vi "AcquisitionInterface1.vi"() -> ()   [LabVIEW 2025]
uses:
  <vilib>/DAQmx/read.llb/DAQmx Read (Analog 1D Wfm NChan NSamp).vi
  <vilib>/Waveform/WDTOps.llb/WDT Append Waveforms DBL.vi
panel:
  out "file path out":path
  in  "file path in":path
  out "error out":errorcluster
  in  "Save to txt":bool
  in  "stop":bool
  out "data":waveform(dbl)[](graph)
  in  "error in":errorcluster
  in  "physical channels":tag
  in  "channel settings":T1={"units"=10348, "input terminal configuration"=-1, "maximum value"=5.0, "minimum value"=-5.0} {"units" items=["Volts"=10348, "From Custom Scale"=10065]; "input terminal configuration" items=["Default"=-1, "RSE"=10083, "NRSE"=10078, "Differential"=10106, "Pseudodifferential"=12529]}
  in  "frequency settings":T2={"frequency (Hz)"=0.001, "number of samples per cycle"=2.0, "number of cycles"=1.0} {"frequency (Hz)" min=0.001 max=100000000.0; "number of samples per cycle" min=2.0 step=1.0; "number of cycles" min=1.0}
  # "Pulsa este botón para que la señal medida se guarde en un archivo .txt"
  # "Ruta en la que se guardará la señal"
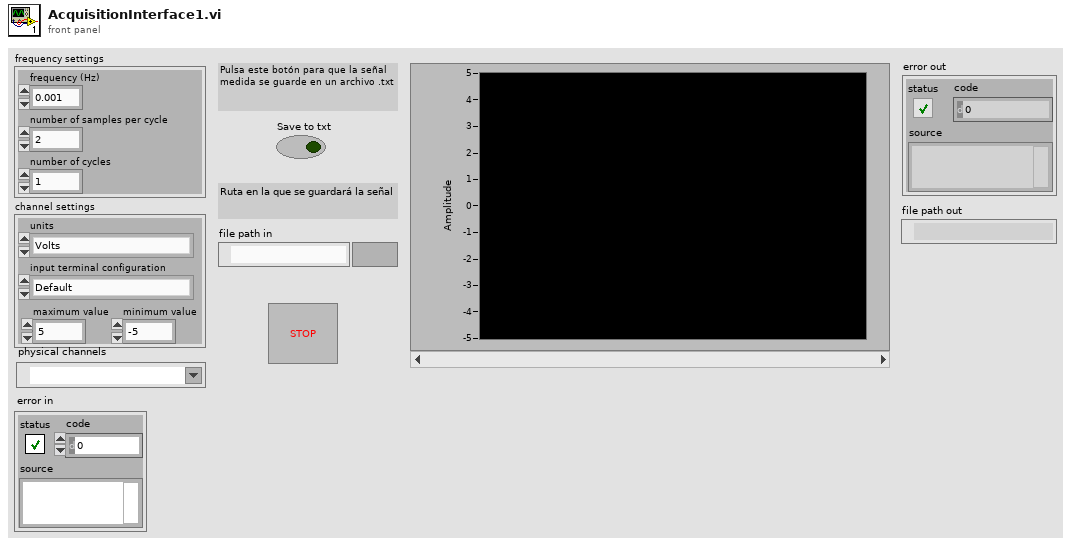
[diagram p1: front panel]
types:
  T1 = cluster{"units":i32, "input terminal configuration":i32, "maximum value":dbl, "minimum value":dbl}
  T2 = cluster{"frequency (Hz)":dbl, "number of samples per cycle":dbl, "number of cycles":dbl}
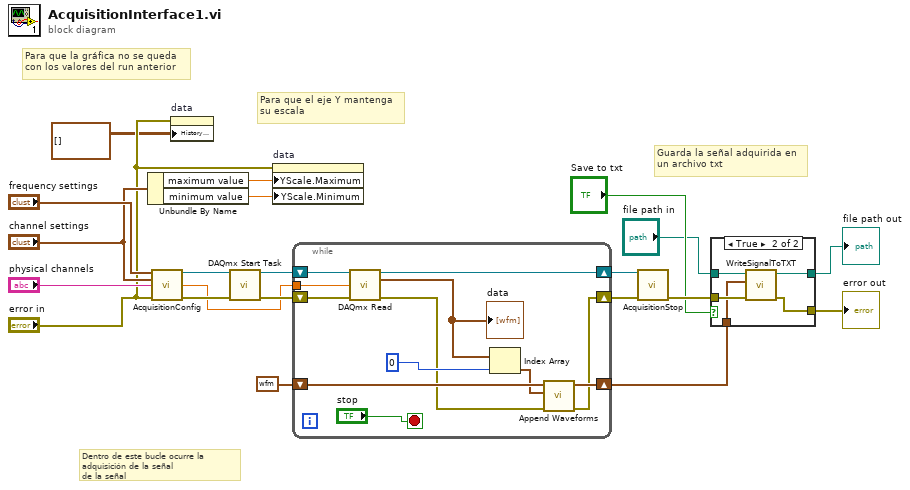
[diagram p0: block diagram]
diagram:
  # "Guarda la señal adquirida en\nun archivo txt"
  # "Dentro de este bucle ocurre la adquisición de la señal\nde la señal"
  # "Para que el eje Y mantenga\nsu escala"
  # "Para que la gráfica no se queda\ncon los valores del run anterior"
  n1 = Unbundle By Name("channel settings") -> ("maximum value"=w12:dbl, "minimum value"=w11:dbl)
  n2 = call "AcquisitionConfig.vi"("frequency settings"="frequency settings", "channel settings"="channel settings", "physical channels"="physical channels", "error in"="error in") -> ("task out"=w18:refnum<k21>, "number of samples"=w8:dbl, "error out"=w19:errorcluster)  [unwired: 9 in]
  n3 = property on="data" class="WFChart (strict)"(error in="error in", "History Data"=waveform(dbl)[][] []) -> ()  [unwired: 1 in, 2 out]
  n4 = call <vilib>:"DAQmx Start Task.vi"("task/channels in"=w18, "error in"=w19) -> ("task out"=w16:refnum<k21>, "error out"=w17:errorcluster)  [unwired: 12 in]
  n5 = property on="data" class="WFChart (strict)"(error in="error in", "YScale.Maximum"=w12, "YScale.Minimum"=w11) -> ()  [unwired: 1 in, 2 out]
  n6 = while {
    tunnel: w8 -> [w31]
    shift-right: [w24] -> w15
    shift-left: w17 -> [w22]
    shift-right: [w32] -> w14
    shift-left: w16 -> [w33]
    shift-right: [w29] -> w5
    shift-left: waveform(dbl) {"t0"=timestamp(0 s since 1904-01-01), "dt"=1.0, "Y"=[]} ("waveform out") -> [w26]
    stop <- "stop" stop-if-true
    n7 = call-poly <vilib>:"DAQmx Read.vi"("task/channels in"=w33, "number of samples per channel"=w31, "error in"=w22) -> ("task out"=w32:refnum<k21>, "data"=w27:waveform(dbl)[], "error out"=w23:errorcluster)  [unwired: 10 in]
    "data" <- w27
    n8 = Index Array(array=w27, index=0) -> (element=w25:waveform(dbl))
    n9 = call-poly <vilib>:"Append Waveforms.vi"("error in (no error)"=w23, "waveform B"=w25, "waveform A"=w26) -> ("error out"=w24:errorcluster, "waveform out"=w29:waveform(dbl))  [unwired: 7 in]
  }
  n10 = call "AcquisitionStop.vi"("task/channels in"=w14, "error in"=w15) -> ("error out"=w6:errorcluster)  [unwired: 13 in]
  n11 = case shown="True" "Save to txt" {
    tunnel: w6 -> [w35 w40]
    tunnel: w5 -> [_ w39]
    tunnel: [w35 w38] -> w3
    tunnel: "file path in" -> [w34 w37]
    tunnel: [w34 w36] -> w1
    frame False {
    }
    frame True {
      n12 = call "WriteSignalToTXT.vi"("error in"=w40, "waveform"=w39, "file path in"=w37) -> ("error out"=w38:errorcluster, "file path out"=w36:path)  [unwired: 7 in]
    }
  }
  "error out" <- w3
  "file path out" <- w1
